vi "Write Element.vi"(8 "error in":errorcluster, 10 "Element":refnum<class "Element.lvclass">, 11 "Structure in":refnum<class "Structure.lvclass">) -> (0 "error out":errorcluster, 3 "Structure out":refnum<class "Structure.lvclass">)   [LabVIEW 2019, in "Structure.lvclass"]
uses:
  Structure.lvclass
  Elements/Element.lvclass
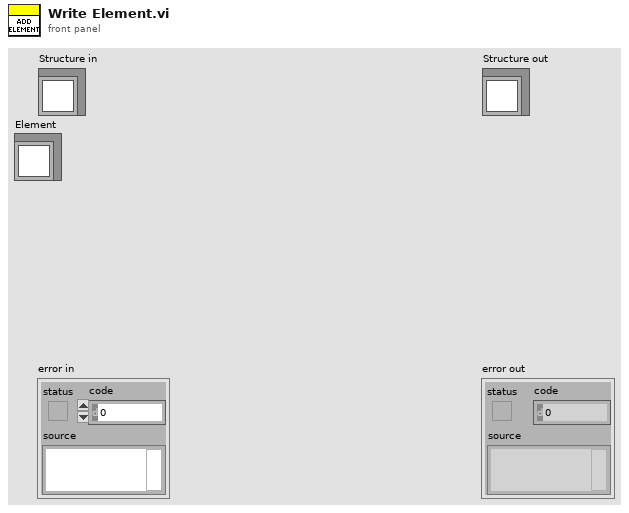
[diagram p1: front panel]
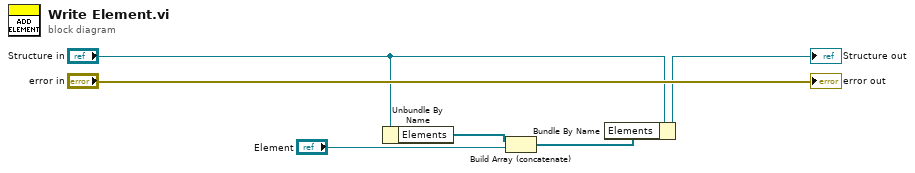
[diagram p0: block diagram]
diagram:
  n1 = Unbundle By Name("Structure in") -> ("Elements"=w3:refnum<class "Element.lvclass">[])
  n2 = Build Array (concatenate)(w3, "Element") -> (w2:refnum<class "Element.lvclass">[])
  n3 = Bundle By Name(cluster="Structure in", "Elements"=w2) -> (→"Structure out":refnum<class "Structure.lvclass">)
  "error out" <- "error in"
